vi "Read Name.vi"(7 "Linked List ID":string, 8 "error in (no error)":errorcluster, 11 "Linked List in":refnum<class "Linked List.lvclass">) -> (0 "error out":errorcluster, 2 "Name":string, 3 "Linked List out":refnum<class "Linked List.lvclass">)   [LabVIEW 2020, in "Linked Lists.lvlib" / "Linked List.lvclass"]
uses:
  <vilib>/gpm_packages/@cs/linked-list/Source/Linked List/Linked List/Linked List.lvclass
  <vilib>/gpm_packages/@cs/linked-list/Source/Linked List/Linked List Definition/Linked List Definition.lvclass
  <vilib>/gpm_packages/@cs/linked-list/Source/Linked List/Linked List/Linked List.lvclass/Linked List.ctl
  <vilib>/gpm_packages/@cs/lookup-table/Source/LookupTable/LookupTable.lvclass/LookupTable.ctl
  13cd71c4-a3bc-4162-8427-a030ade2b40d.vi
  <vilib>/gpm_packages/@cs/lookup-table/Source/LookupTable/Read Table Reference.vi
  13cd71c4-a3bc-4162-8427-a030ade2b40d.vi/5a7267ad-595e-4610-9ac2-8bef780848ff.vi
  <vilib>/gpm_packages/@cs/lookup-table/Source/LookupTable/LookupTable.lvclass
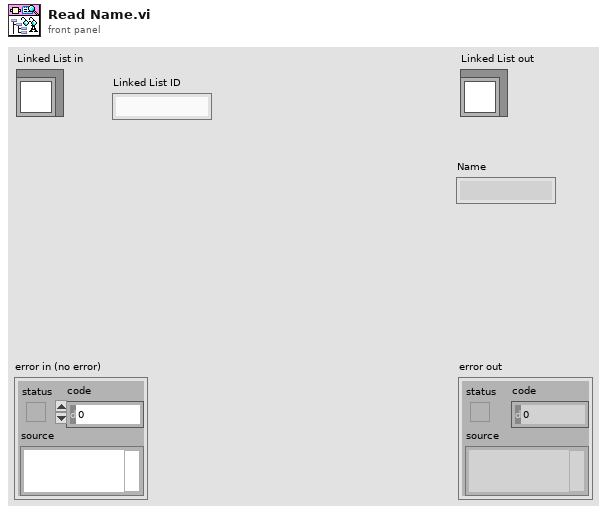
[diagram p1: front panel]
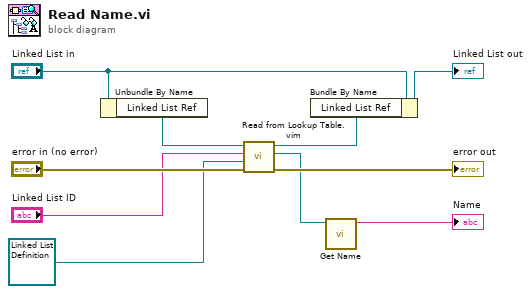
[diagram p0: block diagram]
diagram:
  n1 = Unbundle By Name("Linked List in") -> ("Linked List Ref"=w8:refnum<data-value>)
  n2 = call "Read from Lookup Table.vim"("error in (no error)"="error in (no error)", "Type"=refnum<class "Linked List Definition.lvclass"> refnum ("Linked Lists.lvlib:Linked List Definition.lvclass"), "Item Name"="Linked List ID", "LookupTable Reference"=w8) -> ("error out"=→"error out":errorcluster, "Value"=w2:refnum<class "Linked List Definition.lvclass">, "LookupTable Reference Out"=w5:refnum<data-value>)  [unwired: 4 in, 1 out]
  n3 = Bundle By Name(cluster="Linked List in", "Linked List Ref"=w5) -> (→"Linked List out":refnum<class "Linked List.lvclass">)
  n4 = call <vilib>:"Get Name.vi"("Linked List Definition in"=w2) -> ("Name"=→"Name":string)  [unwired: 8 in, 2 out]
